vi "Read Barometer.vi"(7 "Channel (0: Channel A)":enum16{"Channel A", "Channel B"}(ring), 8 "error in (no error)":errorcluster, 11 "BH Druck PACE Series in":refnum<class "BH Druck PACE Series.lvclass">) -> (0 "error out":errorcluster, 2 "Barometer":dbl format="%#.10g", 3 "BH Druck PACE Series out":refnum<class "BH Druck PACE Series.lvclass">)   [LabVIEW 2022 SP3, in "BH Druck PACE Series.lvclass"]
uses:
  BH Druck PACE Series.lvclass
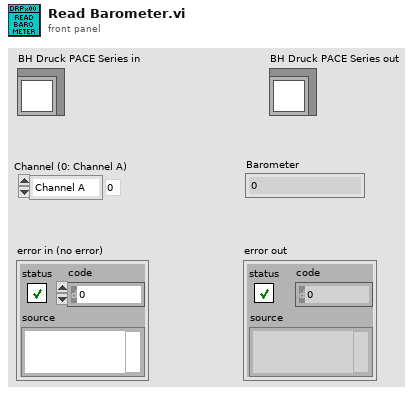
[diagram p1: front panel]
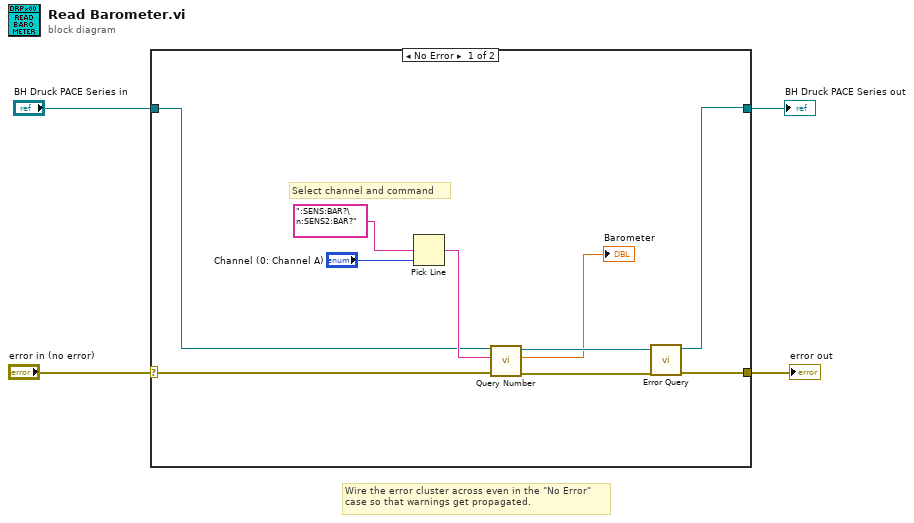
[diagram p0: block diagram]
diagram:
  # "Wire the error cluster across even in the \"No Error\"\ncase so that warnings get propagated."
  n1 = case shown="No Error" "error in (no error)" {
    selector: "error in (no error)" -> [w12 w16]
    tunnel: [w8 w16] -> w3
    tunnel: [w6 w15] -> w1
    tunnel: "BH Druck PACE Series in" -> [w10 w15]
    frame No Error {
      # "Select channel and command"
      n2 = Pick Line(multi-line string=":SENS:BAR?\n:SENS2:BAR?", line index="Channel (0: Channel A)") -> (output string=w11:string)  [unwired: 1 in]
      n3 = call-dynamic "Query Number.vi"("error in (no error)"=w12, "Query String"=w11, "BH Druck PACE Series in"=w10) -> ("error out"=w9:errorcluster, "Numeric Result"=→"Barometer":dbl, "BH Druck PACE Series out"=w7:refnum<class "BH Druck PACE Series.lvclass">)  [unwired: 6 in]
      n4 = call-dynamic "Error Query.vi"("error in (no error)"=w9, "BH Druck PACE Series in"=w7) -> ("error out"=w8:errorcluster, "BH Druck PACE Series out"=w6:refnum<class "BH Druck PACE Series.lvclass">)  [unwired: 8 in]
    }
    frame Error {
    }
  }
  "error out" <- w3
  "BH Druck PACE Series out" <- w1
